vi "题目4.vi"   [LabVIEW 2017]
uses:
  <vilib>/Utility/file.llb/Write Delimited Spreadsheet (DBL).vi
  <vilib>/measure/NI_MABase.lvlib
types:
  T1 = enum16{"open", "replace", "create", "open or create", "replace or create", "replace or create with confirmation"}
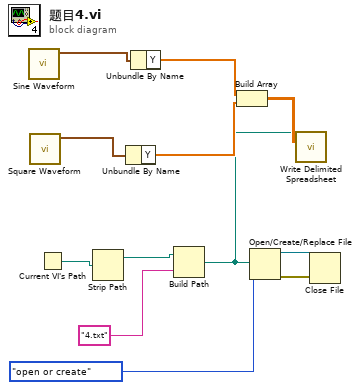
[diagram p0: block diagram]
diagram:
  n1 = call <vilib>:"Sine Waveform.vi"() -> ("signal out"=w12:waveform(dbl))  [unwired: 10 in, 1 out]
  n2 = call <vilib>:"Square Waveform.vi"() -> ("signal out"=w11:waveform(dbl))  [unwired: 10 in, 1 out]
  n3 = Current VI's Path() -> (path=w8:path)
  n4 = Strip Path(path=w8) -> (stripped path=w7:path)  [unwired: 1 out]
  n5 = Unbundle By Name(w11) -> ("Y"=w9:dbl[])
  n6 = Unbundle By Name(w12) -> ("Y"=w10:dbl[])
  n7 = Build Path(base path=w7, name or relative path="4.txt" ("名称或相对路径")) -> (appended path=w3:path)
  n8 = Build Array(w10, w9) -> (w4:dbl[][])
  n9 = Open/Create/Replace File(file path (use dialog)=w3, operation (0:open)=T1."open or create" ("操作(0:open)")) -> (refnum out=w2:refnum<file>, error out=w1:errorcluster)  [unwired: 4 in, 1 out]
  n10 = call-poly <vilib>:"Write Delimited Spreadsheet.vi"("file path (dialog if empty)"=w3, "2D data"=w4) -> ()  [unwired: 12 in, 2 out]
  n11 = Close File(refnum=w2, error in=w1) -> ()  [unwired: 2 out]
